vi "Register HTTP.vi"(8 "error in (no error)":errorcluster, 11 "HTTP Command Bridge in":refnum<class "HTTP Command Bridge.lvclass">) -> (0 "error out":errorcluster, 3 "HTTP Command Bridge out":refnum<class "HTTP Command Bridge.lvclass">)   [LabVIEW 2020, in "Volatus.lvlib" / "HTTP Command Bridge.lvclass"]
uses:
  HTTP Command Bridge.lvclass
  HTTP Command Bridge.lvclass/HTTP Command Bridge.ctl
  Module/Module.lvclass
  VolatusAPI/VolatusAPI.lvclass
  HTTPCmdController/HTTPCmdController.lvclass
  C:/dev/lv20CE/relink/lv-volatus/Volatus/Module/Module.lvclass
  C:/dev/lv20CE/relink/lv-volatus/Volatus/HTTP Command Bridge/HTTP Command Bridge.lvclass
  C:/dev/lv20CE/relink/lv-http-server/HTTP Server/Controller/Controller.lvclass
  C:/dev/lv20CE/relink/lv-http-server/HTTP Server/Handler/Handler.lvclass
  C:/dev/lv20CE/relink/lv-volatus/Volatus/HTTPCmdController/HTTPCmdController.lvclass
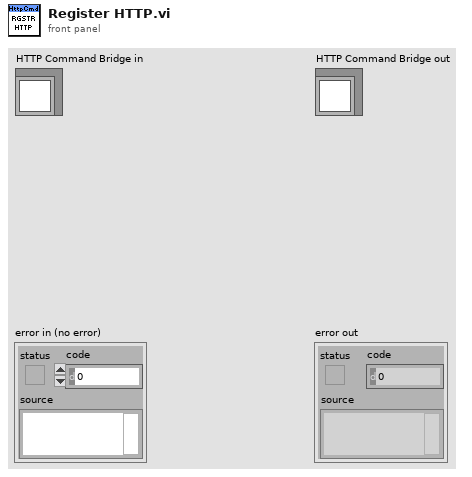
[diagram p1: front panel]
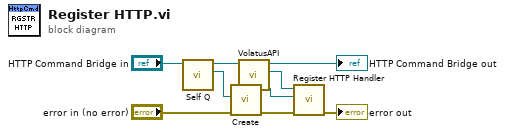
[diagram p0: block diagram]
diagram:
  n1 = call "Self Q.vi"("Module in"="HTTP Command Bridge in") -> ("Self Q"=w1:refnum<class "MessageQ.lvclass">, "Module out"=w2:refnum<class "HTTP Command Bridge.lvclass">)  [unwired: 9 in]
  n2 = call "Create.vi"("error in (no error)"="error in (no error)", "MsgQ"=w1) -> ("error out"=w5:errorcluster, "HTTPCmdController out"=w6:refnum<class "HTTPCmdController.lvclass">)  [unwired: 8 in]
  n3 = call "VolatusAPI.vi"("Module in"=w2) -> ("VolatusAPI"=w7:refnum<class "VolatusAPI.lvclass">, "Module out"=→"HTTP Command Bridge out":refnum<class "HTTP Command Bridge.lvclass">)  [unwired: 9 in]
  n4 = call "Register HTTP Handler.vi"("error in (no error)"=w5, "Handler"=w6, "VolatusAPI in"=w7) -> ("error out"=→"error out":errorcluster)  [unwired: 7 in, 1 out]
